vi "get Plot.vi"(4 "I set":dbl, 5 "Imeas":dbl, 6 "V set":dbl, 7 "Vmeas":dbl, 9 "Iarray":dbl[](array[numeric]), 10 "Varray":dbl[](array[numeric]), 11 "points":u16) -> (0 "logplot":cluster{"Varray manual":dbl[], dbl[]}[](array[cluster]), 3 "Linearplot":T1(array[cluster]))   [LabVIEW 2012]
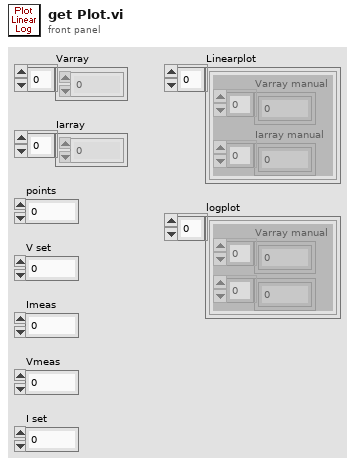
[diagram p1: front panel]
types:
  T1 = cluster{"Varray manual":dbl[], "Iarray manual":dbl[]}[]
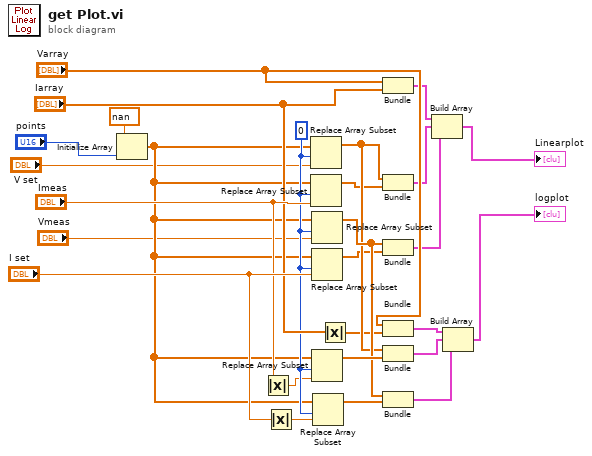
[diagram p0: block diagram]
diagram:
  w19 = 0 ("index")
  n1 = Initialize Array(nan ("element"), "points") -> (w18:dbl[])
  n2 = Absolute Value(x="Imeas") -> (abs(x)=w16:dbl)
  n3 = Absolute Value(x="I set") -> (abs(x)=w20:dbl)
  n4 = Replace Array Subset(array=w18, new element="V set", index=w19) -> (w13:dbl[])
  n5 = Replace Array Subset(array=w18, new element="Imeas", index=w19) -> (w3:dbl[])
  n6 = Replace Array Subset(array=w18, new element="Vmeas", index=w19) -> (w14:dbl[])
  n7 = Replace Array Subset(array=w18, new element="I set", index=w19) -> (w7:dbl[])
  n8 = Replace Array Subset(array=w18, new element=w16, index=w19) -> (w15:dbl[])
  n9 = Replace Array Subset(array=w18, new element=w20, index=w19) -> (w17:dbl[])
  n10 = Absolute Value(x="Iarray") -> (abs(x)=w11:dbl[])
  n11 = Bundle("Varray"="Varray", "Iarray"="Iarray") -> (w6:cluster{"Varray":dbl[], "Iarray":dbl[]})  [unwired: 1 in]
  n12 = Bundle(w13, w3) -> (w5:cluster{dbl[], dbl[]})  [unwired: 1 in]
  n13 = Bundle(w14, w7) -> (w8:cluster{dbl[], dbl[]})  [unwired: 1 in]
  n14 = Bundle("Varray"="Varray", w11) -> (w21:cluster{"Varray":dbl[], dbl[]})  [unwired: 1 in]
  n15 = Bundle(w13, w15) -> (w22:cluster{dbl[], dbl[]})  [unwired: 1 in]
  n16 = Bundle(w14, w17) -> (w23:cluster{dbl[], dbl[]})  [unwired: 1 in]
  n17 = Build Array(w6, w5, w8) -> (→"Linearplot":cluster{"Varray":dbl[], "Iarray":dbl[]}[])
  n18 = Build Array(w21, w22, w23) -> (→"logplot":cluster{"Varray":dbl[], dbl[]}[])
